vi "WriteSizeMat_2DArray_FXP.vi"(6 "Channel":i32=1, 8 "error in":errorcluster, 9 "Height":i32, 10 "Width":i32, 11 "Array in":fxp<+/-,8,8>[][](array[numeric])) -> (0 "error out":errorcluster, 3 "Array out":fxp<+/-,8,8>[][](array[numeric]))   [LabVIEW 2020, in "OpenLvVision_OpenCv.lvlib"]
doc: "Write size of the datatype\nNo malleable to breake vi inlining!"
uses:
  OpenLvVision_OpenCv.lvlib
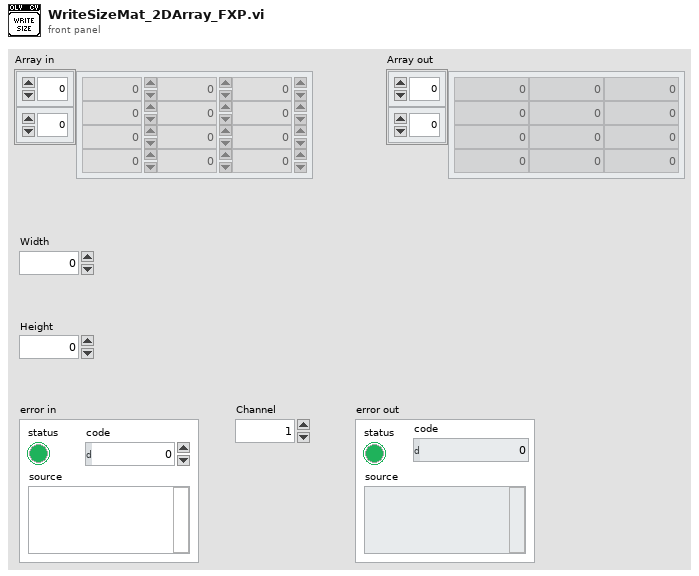
[diagram p1: front panel]
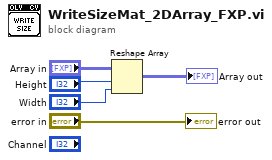
[diagram p0: block diagram]
diagram:
  n1 = Reshape Array("Array in", "Height", "Width") -> (→"Array out":fxp<+/-,8,8>[][])
  "error out" <- "error in"
